vi "Global_CMD_Data In.vi"() -> ()   [LabVIEW 2020, in "GameController_SEN.lvlib"]
uses:
  GameController_SEN.lvlib
  Shared Code/TypeDefs/ENUM_Controller Buzz Select.ctl
panel:
  in  "CMD_SEN_GameController_BUZZNumber":dbl
  in  "CMD_SEN_GameController_BUZZ Select":T1
  # "The Names of the Data items in the Global Variable MUST describe who the Single Writer is\nFor Command Globals the Commander(CMD) represents Teleop or Autonomous or other command loop.\nThe naming convention for a Command Actuator Global is:   \n\nCMD_ACT_SubSystem_Data Name\n\nExample:\nCMD_ACT_Drive_Data\nCMD_ACT_Hopper_Eject Ball"
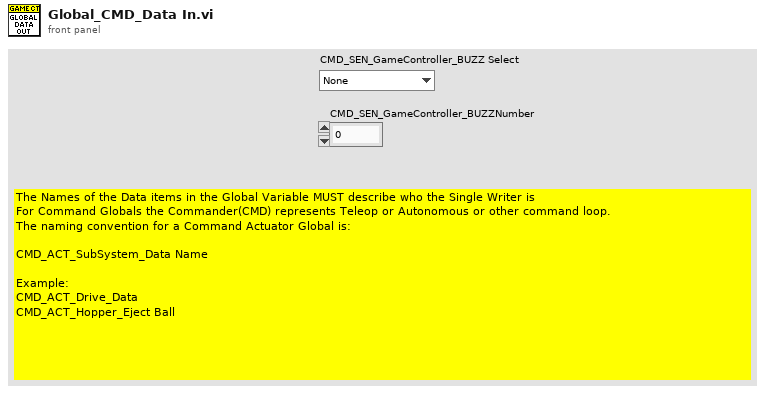
[diagram p1: front panel]
types:
  T1 = typedef "ENUM_Controller Buzz Select.ctl" = enum16{"None", "Timed Full ON", "Set Intensity", ".5 Sec Cycle Count"}
diagram:
